vi "TemperatureController main.vi"(8 "Supervising module":T1, 11 "Controller module":T2) -> ()   [LabVIEW 2024, in "Temperature controller.lvlib"]
doc: "Heater names:\nVTI space [K]\nSample [K]\nHeater3 [K]\nHeater4 [K]\n\n\" Initialize: Visa resource name (VISA session) / Instrument model number (string)\n\" Update: - / TC sensors {VTI space, Sample, He pot, Trap, Ambient, SetP_VTI, SetP_Smp, SetP_Pot, SetP_Trap, Range out 1, Out 1, Out 2} (numeric cluster)\n\" Set temperature: Set temperature {VTI space, Sample, Heater 3, Heater 4, Out 1, Out 2, Range out 1} (numeric cluster) / Set temperature {VTI space, Sample, Heater 3, Heater 4, Out 1, Out 2, Range out 1} (numeric cluster)\n\" Set point: Set point {Heater, Tmp} (cluster: string, numeric) / Set point {Heater, Tmp} (cluster: string, numeric)\n\" End: - / -\n\" Disconnect: - / -"
uses:
  Temperature controller.lvlib
  Messenger service/Data types/Modul ref.ctl
  Messenger service/Data types/Mailbox address.ctl
  Messenger service/Data types/Module name.ctl
  ctl/Set temperature.ctl
  ctl/Set point.ctl
  ctl/MSG for VTI.ctl
  ctl/TC commands.ctl
  <instrlib>/Lake Shore 350/Lake Shore 350.lvlib
  Messenger service/MessengerLib.lvlib
panel:
  out "Ended":bool
  out "TC port":refnum<visa-resource-name>
  out "Conected":bool
  # "Controls"
  # "Indicators"
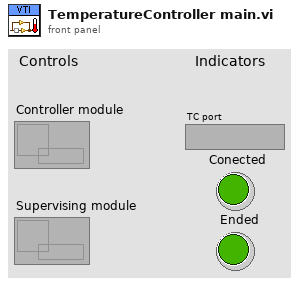
[diagram p1: front panel]
types:
  T1 = typedef "MessengerLib.lvlib/Mailbox address.ctl" = refnum<queue>
  T2 = typedef "MessengerLib.lvlib/Modul ref.ctl" = refnum<queue>
  T3 = typedef "Temperature controller.lvlib/MSG for VTI.ctl" = cluster{"Command":T4, "Data":variant}
  T4 = typedef "Temperature controller.lvlib/TC commands.ctl" = enum16{"Initialize", "Update", "Stop tmp change", "Set temperature", "Set point", "Disconnect", "End", "Ignore"}
  T5 = typedef "Module name.ctl" = enum16{"Emty", "Magnet", "VTI", "Excitation", "Servo", "Acquisition", "Rotator", "Digitizer", "SMU2450", "Carousel", "Multimeter", "Tmp monitor", "Power monitor"}
  T6 = cluster{"Baud Rate":u32, "Parity":u16, "Data Bits":u16, "Stop Bits":u16, "Flow Control":u16}
  T7 = typedef "Temperature controller.lvlib/Set temperature.ctl" = cluster{"VTI space [K]":dbl, "Sample [K]":dbl, "Heater3 [K]":dbl, "Heater4 [K]":dbl, "Out 1 [%]":dbl, "Out 2 [%]":dbl, "Range out 1":u16}
  T8 = typedef "Temperature controller.lvlib/Set point.ctl" = cluster{"Heater":string, "Tmp [K]":dbl}
  T9 = typedef "Temperature controller.lvlib/TC sensors.ctl" = cluster{"VTI space":dbl, "Sample":dbl, "He pot":dbl, "Trap":dbl, "Ambient":dbl, "SetP_VTI":dbl, "SetP_Smp":dbl, "SetP_Pot":dbl, "SetP_Trap":dbl, "Range out 1":u16, "Out 1 [%]":dbl, "Out 2 [%]":dbl}
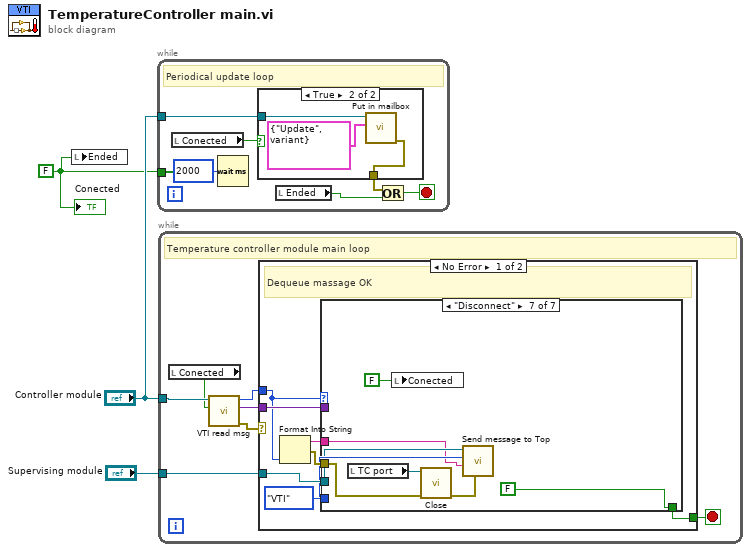
[diagram p0: block diagram]
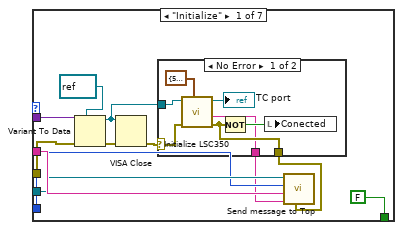
[diagram p3: hidden frame]
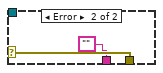
[diagram p4: hidden frame]
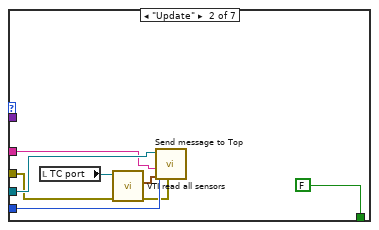
[diagram p5: hidden frame]
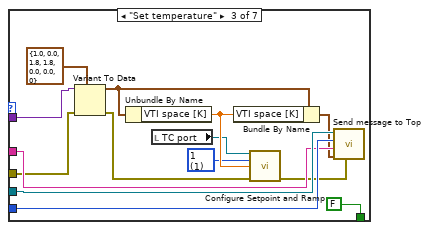
[diagram p6: hidden frame]
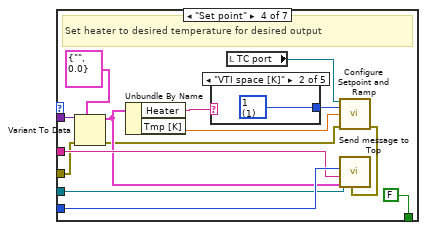
[diagram p7: hidden frame]
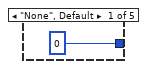
[diagram p8: hidden frame]
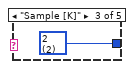
[diagram p9: hidden frame]
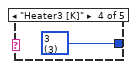
[diagram p10: hidden frame]
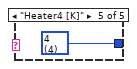
[diagram p11: hidden frame]
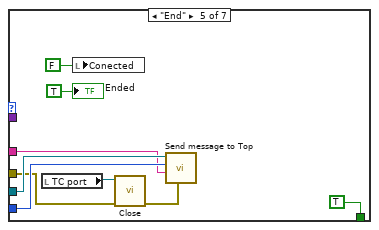
[diagram p12: hidden frame]
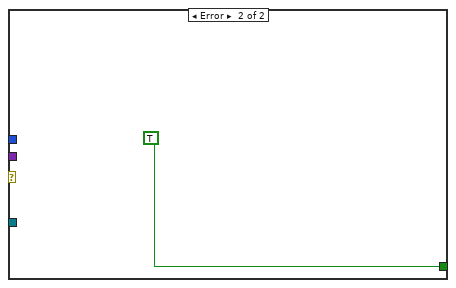
[diagram p14: hidden frame]
diagram:
  w1 = FALSE ("Initialized?")
  n1 = local write "Ended"(w1) -> ()
  n2 = while "Periodical update loop" {
    tunnel: "Controller module" -> [w7]
    tunnel: w1 -> [_]
    stop <- w5 stop-if-true
    # "Periodical update loop"
    n3 = local read "Conected"() -> (w8:bool)
    n4 = Wait (ms)(milliseconds to wait=u32 2000) -> ()  [unwired: 1 out]
    n5 = case shown="True" w8 {
      tunnel: w7 -> [_ w12]
      tunnel: [_ w10] -> w4
      frame False {
      }
      frame True {
        n6 = call "Put in mailbox.vi"("Message"=T3 {"Command"=enum."Update", "Data"=variant}, "Queue in"=w12) -> ("error out"=w10:errorcluster)  [unwired: 7 in, 2 out]
      }
    }
    n7 = local read "Ended"() -> (w6:bool)
    n8 = Or(x=w4, y=w6) -> (x .or. y?=w5:bool)
  }
  n9 = while {
    tunnel: "Controller module" -> [w18]
    tunnel: "Supervising module" -> [w19]
    stop <- w14 stop-if-true
    # "Temperature controller module main loop"
    n10 = local read "Conected"() -> (w17:bool)
    n11 = call "VTI read msg.vi"("Initialized?"=w17, "Queue in"=w18) -> ("error out"=w13:errorcluster, "Data"=w16:variant, "Command"=w15:T4)  [unwired: 6 in, 1 out]
    n12 = case shown="No Error" w13 {
      tunnel: w19 -> [w25 _]
      tunnel: w16 -> [w24 _]
      tunnel: w15 -> [w22 _]
      tunnel: [w20 TRUE] -> w14
      frame No Error {
        # "Dequeue massage OK"
        n13 = Format Into String(w22) -> (resulting string=w23:string, error out=w21:errorcluster)  [unwired: 3 in]
        n14 = case shown="\"Disconnect\"" w22 {
          tunnel: Module_name."VTI" ("Module name") -> [w33 w55 w69 w83 w97 _ w105]
          tunnel: w25 -> [w34 w54 w68 w82 w95 _ w103]
          tunnel: w24 -> [w37 _ w66 w80 _ _ _]
          tunnel: w23 -> [w35 w50 w67 w81 w94 _ w102]
          tunnel: w21 -> [w36 w52 w64 w79 w92 _ w100]
          tunnel: [FALSE FALSE FALSE FALSE TRUE _ FALSE] -> w20
          frame "Initialize" {
            n15 = Variant To Data(error in=w36, type=refnum<visa-resource-name> refnum ("VISA resource name"), Variant=w37) -> (data=w28:refnum<visa-resource-name>, error out=w29:errorcluster)
            n16 = VISA Close(VISA resource name=w28, error in (no error)=w29) -> (error out=w30:errorcluster)
            n17 = case shown="No Error" w30 {
              selector: w30 -> [w39 w47]
              tunnel: [w42 w47] -> w31
              tunnel: [w41 ""] -> w32
              tunnel: w28 -> [w40 _]
              frame No Error {
                n18 = call "Initialize LSC350.vi"("Serial Configuration"=T6 {"Baud Rate"=57600, "Parity"=1, "Data Bits"=7, "Stop Bits"=10, "Flow Control"=0}, "error in (no error)"=w39, "VISA resource name"=w40) -> ("error out"=w42:errorcluster, "Instrument Model Number"=w41:string, "VISA resource name out"=→"TC port":refnum<visa-resource-name>)  [unwired: 6 in]
                n19 = Not(x=w42) -> (.not. x?=w43:bool)
                n20 = local write "Conected"(w43) -> ()
              }
              frame Error {
              }
            }
            n21 = call "Send message to Top.vi"("Error in (no error)"=w31, "Data"=w32, "Response"=w35, "Module"=w33, "Mailbox address in"=w34) -> ()  [unwired: 5 in, 2 out]
          }
          frame "Update" {
            n22 = local read "TC port"() -> (w53:refnum<visa-resource-name>)
            n23 = call "VTI read all sensors.vi"("error in (no error)"=w52, "VISA Refnum in"=w53) -> ("error out"=w51:errorcluster, "TC sensors [K]"=w49:T9)  [unwired: 7 in, 1 out]
            n24 = call "Send message to Top.vi"("Error in (no error)"=w51, "Data"=w49, "Response"=w50, "Module"=w55, "Mailbox address in"=w54) -> ()  [unwired: 5 in, 2 out]
          }
          frame "Set temperature" {
            w57 = u16 1 items=["1"=1, "2"=2, "3"=3, "4"=4] ("Output's Control Loop (1:1)")
            n25 = Variant To Data(error in=w64, type=T7 {"VTI space [K]"=1.0, "Sample [K]"=0.0, "Heater3 [K]"=1.8, "Heater4 [K]"=1.8, "Out 1 [%]"=0.0, "Out 2 [%]"=0.0, "Range out 1"=0}, Variant=w66) -> (data=w63:T7, error out=w59:errorcluster)
            n26 = Unbundle By Name(w63) -> ("VTI space [K]"=w60:dbl)
            n27 = local read "TC port"() -> (w58:refnum<visa-resource-name>)
            n28 = Bundle By Name(cluster=w63, "VTI space [K]"=w60) -> (w62:T7)
            n29 = call <instrlib>:"Configure Setpoint and Ramp.vi"("VISA resource name"=w58, "Output's Control Loop (1:1)"=w57, "Setpoint (0.00000)"=w60, "error in (no error)"=w59) -> ("error out"=w61:errorcluster)  [unwired: 10 in, 1 out]
            n30 = call "Send message to Top.vi"("Error in (no error)"=w61, "Data"=w62, "Response"=w67, "Module"=w69, "Mailbox address in"=w68) -> ()  [unwired: 5 in, 2 out]
          }
          frame "Set point" {
            # "Set heater to desired temperature for desired output"
            n31 = Variant To Data(error in=w79, type=T8 {"Heater"="", "Tmp [K]"=0.0}, Variant=w80) -> (data=w75:T8, error out=w73:errorcluster)
            n32 = Unbundle By Name(w75) -> ("Heater"=w76:string, "Tmp [K]"=w71:dbl)
            n33 = case shown="\"VTI space [K]\"" w76 {
              tunnel: [u16 0 ("Output's Control Loop (1:1)") w85 w86 w87 w88] -> w74
              frame "None", Default {
              }
              frame "VTI space [K]" {
                w85 = u16 1 items=["1"=1, "2"=2, "3"=3, "4"=4] ("Output's Control Loop (1:1)")
              }
              frame "Sample [K]" {
                w86 = u16 2 items=["1"=1, "2"=2, "3"=3, "4"=4] ("Output's Control Loop (1:1)")
              }
              frame "Heater3 [K]" {
                w87 = u16 3 items=["1"=1, "2"=2, "3"=3, "4"=4] ("Output's Control Loop (1:1)")
              }
              frame "Heater4 [K]" {
                w88 = u16 4 items=["1"=1, "2"=2, "3"=3, "4"=4] ("Output's Control Loop (1:1)")
              }
            }
            n34 = local read "TC port"() -> (w72:refnum<visa-resource-name>)
            n35 = call <instrlib>:"Configure Setpoint and Ramp.vi"("VISA resource name"=w72, "Output's Control Loop (1:1)"=w74, "Setpoint (0.00000)"=w71, "error in (no error)"=w73) -> ("error out"=w78:errorcluster)  [unwired: 10 in, 1 out]
            n36 = call "Send message to Top.vi"("Error in (no error)"=w78, "Data"=w75, "Response"=w81, "Module"=w83, "Mailbox address in"=w82) -> ()  [unwired: 5 in, 2 out]
          }
          frame "End" {
            n37 = local read "TC port"() -> (w93:refnum<visa-resource-name>)
            n38 = local write "Conected"(FALSE ("Initialized?")) -> ()
            n39 = call <instrlib>:"Close.vi"("error in (no error)"=w92, "VISA resource name"=w93) -> ("error out"=w96:errorcluster)  [unwired: 9 in]
            n40 = call "Send message to Top.vi"("Error in (no error)"=w96, "Response"=w94, "Module"=w97, "Mailbox address in"=w95) -> ()  [unwired: 6 in, 2 out]
            "Ended" <- TRUE ("Initialized?")
          }
          frame "Ignore", Default {
          }
          frame "Disconnect" {
            n41 = local read "TC port"() -> (w101:refnum<visa-resource-name>)
            n42 = local write "Conected"(FALSE ("Initialized?")) -> ()
            n43 = call <instrlib>:"Close.vi"("error in (no error)"=w100, "VISA resource name"=w101) -> ("error out"=w104:errorcluster)  [unwired: 9 in]
            n44 = call "Send message to Top.vi"("Error in (no error)"=w104, "Response"=w102, "Module"=w105, "Mailbox address in"=w103) -> ()  [unwired: 6 in, 2 out]
          }
        }
      }
      frame Error {
      }
    }
  }
  "Conected" <- w1
